vi "test_generic.vi"() -> ()   [LabVIEW 2017, in "GenericAnalyser.lvclass"]
uses:
  GenericAnalyser.lvclass
  main/labview_source/type_definitions/clusters/controls_refs.ctl
  common/classes/Image/Image/Image.lvclass
  common/classes/GenericComponent/GenericComponent/GenericComponent.lvclass
  common/classes/ErrorController/ErrorController/ErrorController.lvclass
  common/classes/GenericToplevelComponent/GenericToplevelComponent/common_trigger_enum.ctl
  common/classes/GenericToplevelComponent/GenericToplevelComponent/GenericToplevelComponent.lvclass
panel:
  out "error loaded?":bool
  in  "start button":bool
  in  "number of channels":i32=1
  in  "send image button":bool
  in  "stop":bool
  in  "create button":bool
  # "Test VI for Analyser components"
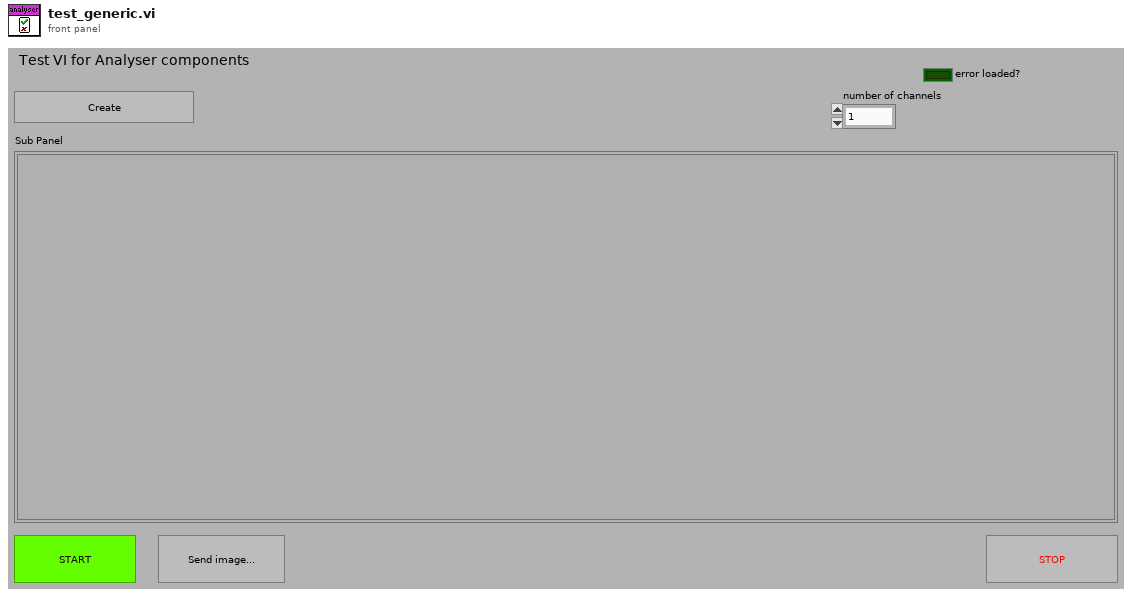
[diagram p1: front panel]
types:
  T1 = typedef "controls_refs.ctl" = cluster{"buttons":cluster{"start_focus":refnum<vi>, "start_single_sweep":refnum<vi>, "start_experiment":refnum<vi>, "save":refnum<vi>, "exit":refnum<vi>}, "tabs":cluster{"main":refnum<vi>, "settings":refnum<vi>}, "subpanels":cluster{"imagingMode":refnum<vi>, "scanHead":refnum<vi>, "display":refnum<vi>, "experimentController":refnum<vi>, "instrument":refnum<vi>, "stage":refnum<vi>, "stimulator":refnum<vi>, "dataCollection":refnum<vi>, "analyser":refnum<vi>, "daq":refnum<vi>, "imageAssembler":refnum<vi>}, "drop-downs":cluster{"imagingMode":refnum<vi>, "experimentalController":refnum<vi>, "objective":refnum<vi>}, "status lights":cluster{"experimentController":refnum<vi>, "imagingMode":refnum<vi>, "scanHead":refnum<vi>, "daq":refnum<vi>, "imageAssembler":refnum<vi>, "dataCollection":refnum<vi>, "display":refnum<vi>, "analyser":refnum<vi>, "stage":refnum<vi>, "stimulator":refnum<vi>, "instrument":refnum<vi>}, "message":refnum<vi>, "stimulator enabled?":refnum<vi>, "saving":cluster{"data folder path":refnum<vi>, "file base name":refnum<vi>, "notebook":refnum<vi>}, "progress bar":refnum<vi>, "update icon":refnum<vi>, "title":refnum<vi>, "main vi":refnum<vi>, "user":refnum<vi>}
  T2 = typedef "GenericToplevelComponent.lvclass/common_trigger_enum.ctl" = enum16{"NULL", "initialise", "terminate", "fetch command", "fetch data", "attach observer", "register as observer", "detach observer", "acknowledge", "start", "stop", "sweep started", "sweep finished", "experiment started", "experiment stopped"}
  T3 = typedef "XComponentSpecification.xctl/data.ctl" = cluster{"class path":string, "configuration":string, "label":string, "settings name":string}
  T4 = typedef "Image Type" = u32
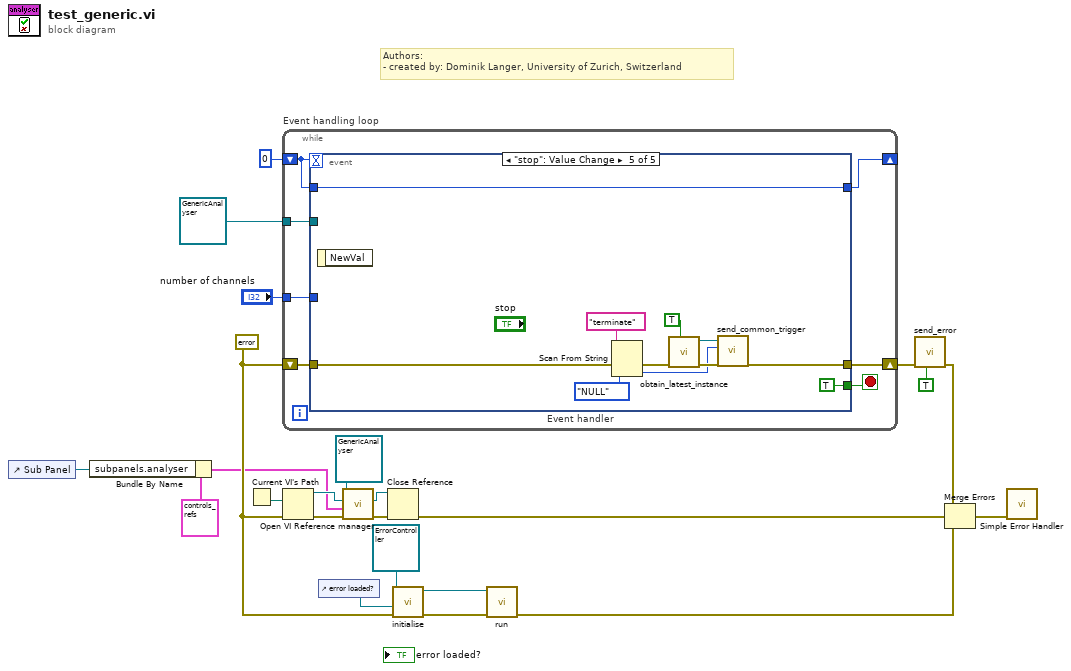
[diagram p0: block diagram]
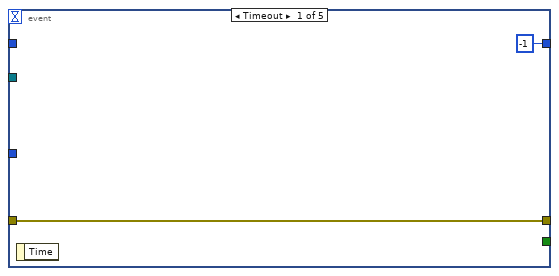
[diagram p2: hidden frame]
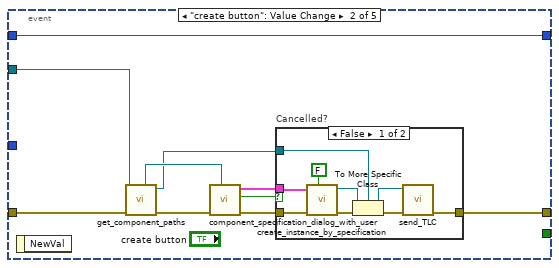
[diagram p3: hidden frame]
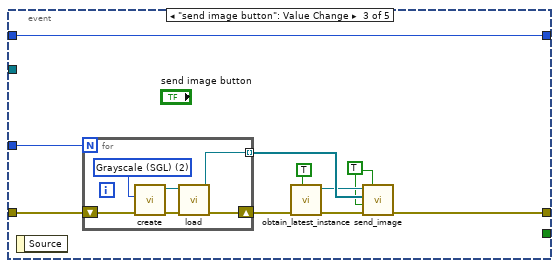
[diagram p5: hidden frame]
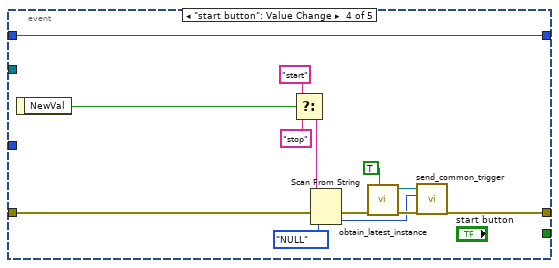
[diagram p6: hidden frame]
diagram:
  w8 = errorcluster {"status"=FALSE, "code"=0, "source"=""} ("error in (no error)")
  # "Authors: \n- created by: Dominik Langer, University of Zurich, Switzerland"
  n1 = control-ref of="Sub Panel"() -> (w19:refnum<vi>)
  n2 = Bundle By Name(cluster=T1 {"buttons"={"start_focus"=refnum, "start_single_sweep"=refnum, "start_experiment"=refnum, "save"=refnum, "exit"=refnum}, "tabs"={"main"=refnum, "settings"=refnum}, "subpanels"={"imagingMode"=refnum, "scanHead"=refnum, "display"=refnum, "experimentController"=refnum, "instrument"=refnum, "stage"=refnum, "stimulator"=refnum, "dataCollection"=refnum, "analyser"=refnum, "daq"=refnum, "imageAssembler"=refnum}, "drop-downs"={"imagingMode"=refnum, "experimentalController"=refnum, "objective"=refnum}, "status lights"={"experimentController"=refnum, "imagingMode"=refnum, "scanHead"=refnum, "daq"=refnum, "imageAssembler"=refnum, "dataCollection"=refnum, "display"=refnum, "analyser"=refnum, "stage"=refnum, "stimulator"=refnum, "instrument"=refnum}, "message"=refnum, "stimulator enabled?"=refnum, "saving"={"data folder path"=refnum, "file base name"=refnum, "notebook"=refnum}, "progress bar"=refnum, "update icon"=refnum, "title"=refnum, "main vi"=refnum, "user"=refnum} ("control references"), "subpanels.analyser"=w19) -> (w3:T1)
  n3 = Current VI's Path() -> (path=w21:path)
  n4 = while "Event handling loop" {
    shift-right: [w29] -> w10
    shift-left: w8 -> [w30]
    shift-right: [w27] -> _
    shift-left: 0 -> [w28]
    tunnel: "number of channels" -> [w25]
    tunnel: refnum<class "GenericAnalyser.lvclass"> refnum ("GeneralAnalyser.lvclass") -> [w24]
    stop <- w26 stop-if-true
    n5 = event "Event handler" shown="[4] \"stop\": Value Change" {
      selector: _ -> [_ _ _ _ _]
      dyn-events: _ -> [_ _ _ _ _]
      timeout: w28 -> [_ _ _ _ _]
      tunnel: w30 -> [w31 w34 w61 w75 w87]
      tunnel: [w31 w41 w57 w79 w90] -> w29
      tunnel: [-1 w42 w62 w81 w92] -> w27
      tunnel: w28 -> [_ w42 w62 w81 w92]
      tunnel: [_ _ _ _ TRUE] -> w26
      tunnel: w25 -> [_ _ w59 _ _]
      tunnel: w24 -> [_ w36 _ _ _]
      event Timeout {
        n6 = event-data() -> ()  [unwired: 2 out]
      }
      event "create button": Value Change {
        n7 = event-data() -> ()  [unwired: 2 out]
        n8 = call-dynamic "get_component_paths.vi"("error in (no error)"=w34, "GenericComponent in"=w36) -> ("error out"=w33:errorcluster, "GenericComponent out"=w35:refnum<class "GenericAnalyser.lvclass">, "component type directory"=w37:path)  [unwired: 4 in, 3 out]
        n9 = call "component_specification_dialog_with_user.vi"("start path"=w37, "error in (no error)"=w33) -> ("error out"=w40:errorcluster, "cancelled?"=w38:bool, "component specification out"=w39:T3)  [unwired: 7 in]
        n10 = case "Cancelled?" shown="False" w38 {
          tunnel: [w51 w52] -> w41
          tunnel: w35 -> [w50 _]
          tunnel: w40 -> [w45 w52]
          tunnel: w39 -> [w44 _]
          frame False {
            n11 = call "create_instance_by_specification.vi"("call constructor?"=FALSE, "error in (no error)"=w45, "component specification"=w44) -> ("error out"=w49:errorcluster, "GenericPlugin out"=w48:refnum<class "GenericComponent.lvclass">)  [unwired: 6 in, 1 out]
            n12 = To More Specific Class(target class=w50, reference=w48, error in=w49) -> (specific class reference=w46:refnum<class "GenericAnalyser.lvclass">, error out=w47:errorcluster)
            n13 = call-dynamic "send_TLC.vi"("error in (no error)"=w47, "GenericToplevelComponent in"=w46) -> ("error out"=w51:errorcluster)  [unwired: 9 out]
          }
          frame True {
          }
        }
      }
      event "send image button": Value Change {
        w53 = TRUE ("image finished?")
        n14 = event-data() -> ()  [unwired: 2 out]
        n15 = for {
          N: w59 -> [_]
          shift-right: [w66] -> w60
          shift-left: w61 -> [w68]
          tunnel: [w63] -> w55 mode=indexing
          w64 = T4 2 items=["Grayscale (U8)", "Grayscale (I16)", "Grayscale (SGL)", "Complex (CSG)", "RGB (U32)", "HSL (U32)", "RGB (U64)", "Grayscale (U16)"] ("Image Type")
          n16 = call "create.vi"("error in (no error)"=w68, "Image Type"=w64) -> ("error out"=w67:errorcluster, "Image out"=w65:refnum<class "Image.lvclass">)  [unwired: 2 in, 6 out]
          n17 = call-dynamic "load.vi"("error in (no error)"=w67, "Image in"=w65) -> ("error out"=w66:errorcluster, "Image out"=w63:refnum<class "Image.lvclass">)  [unwired: 2 in, 6 out]
        }
        n18 = call "obtain_latest_instance.vi"("quick, but maybe outdated?"=TRUE, "error in (no error)"=w60) -> ("error out"=w56:errorcluster, "GeneralAnalyser out"=w54:refnum<class "GenericAnalyser.lvclass">)  [unwired: 8 out]
        n19 = call-dynamic "send_image.vi"("force sending?"=w53, "error in (no error)"=w56, "image finished?"=w53, "image (channels)"=w55, "GenericToplevelComponent in"=w54) -> ("error out"=w57:errorcluster)  [unwired: 4 in, 2 out]
      }
      event "start button": Value Change {
        n20 = event-data() -> ("NewVal"=w76:bool)  [unwired: 1 out]
        n21 = Select(t="start", s=w76, f="stop") -> (s? t:f=w71:string)
        n22 = Scan From String(input string=w71, error in=w75, default 1=common_trigger_enum."NULL" ("f")) -> (error out=w74:errorcluster, output 1=w70:T2)  [unwired: 2 in, 2 out]
        n23 = call "obtain_latest_instance.vi"("quick, but maybe outdated?"=TRUE, "error in (no error)"=w74) -> ("error out"=w80:errorcluster, "GeneralAnalyser out"=w77:refnum<class "GenericAnalyser.lvclass">)  [unwired: 8 out]
        n24 = call-dynamic "send_common_trigger.vi"("error in (no error)"=w80, "trigger"=w70, "GenericToplevelComponent in"=w77) -> ("error out"=w79:errorcluster)  [unwired: 6 in, 2 out]
      }
      event "stop": Value Change {
        n25 = event-data() -> ()  [unwired: 2 out]
        n26 = Scan From String(input string="terminate", error in=w87, default 1=common_trigger_enum."NULL" ("f")) -> (error out=w86:errorcluster, output 1=w84:T2)  [unwired: 2 in, 2 out]
        n27 = call "obtain_latest_instance.vi"("quick, but maybe outdated?"=TRUE, "error in (no error)"=w86) -> ("error out"=w91:errorcluster, "GeneralAnalyser out"=w88:refnum<class "GenericAnalyser.lvclass">)  [unwired: 8 out]
        n28 = call-dynamic "send_common_trigger.vi"("error in (no error)"=w91, "trigger"=w84, "GenericToplevelComponent in"=w88) -> ("error out"=w90:errorcluster)  [unwired: 6 in, 2 out]
      }
    }
  }
  n29 = Open VI Reference(vi path=w21, error in (no error)=w8) -> (vi reference=w4:refnum<vi>, error out=w6:errorcluster)  [unwired: 4 out]
  n30 = control-ref of="error loaded?"() -> (w14:refnum<vi>)
  n31 = call-dynamic "manager.vi"("error in (no error)"=w6, "control references"=w3, "top-level VI ref in"=w4, "GenericToplevelComponent in"=refnum<class "GenericAnalyser.lvclass"> refnum ("GenericAnalyser.lvclass")) -> ("error out"=w5:errorcluster, "top-level VI ref out"=w2:refnum<vi>)  [unwired: 5 in, 1 out]
  n32 = Close Reference(reference=w2, error in (no error)=w5) -> (error out=w17:errorcluster)
  n33 = call-dynamic "initialise.vi"("error in (no error)"=w8, "error boolean"=w14, "ErrorController in"=refnum<class "ErrorController.lvclass"> refnum ("ErrorController.lvclass")) -> ("error out"=w16:errorcluster, "ErrorController out"=w15:refnum<class "ErrorController.lvclass">)  [unwired: 7 in]
  n34 = call "run.vi"("error in (no error)"=w16, "ErrorController in"=w15) -> ("error out"=w12:errorcluster)  [unwired: 8 in, 1 out]
  n35 = call "send_error.vi"("last error? (F)"=TRUE, "error in (no error)"=w10) -> ("error out"=w9:errorcluster)  [unwired: 9 in]
  n36 = Merge Errors(w9, w17, w12) -> (w22:errorcluster)
  n37 = call <vilib>:"Simple Error Handler.vi"("error in (no error)"=w22) -> ()  [unwired: 1 in, 8 out]
